vi "cluster_append.vi"(0 "magnitude value":dbl, 1 "phase value":dbl, 2 "Tx FFT mag":dbl, 3 "Tx FFT phase":dbl, 4 "shift value":dbl, 5 "Input Cluster":T1={"Magnitude meas."=[], "Phase meas."=[], "Shift meas."=[], "cw"=TRUE, "projections per image"=0, "ramp-up readouts"=0, "current sense type"="", "Number of pulses per image"=0, "Rotation enabled"=TRUE, "Rotary position"=[], "Baseline magnitude"=0.0, "Baseline phase"=0.0, "Wait readouts"=0, "Shift waveform type"="", "Shift enabled"=TRUE, "Time domain data"=[], "Motor pulse duration"=0.0, "Shift Amp pk"=0.0, "Shift DC offset"=0.0, "Notes"="", "Reconstructed image"=bytes[0], "Rotary encoder type"="", "Image start"=timestamp(0 s since 1904-01-01), "Image stop"=timestamp(0 s since 1904-01-01), "readouts per projection"=0, "Recon enabled"=FALSE, "Bidirectional shift"=FALSE, "Imager mode"="", "Shift delay"=0.0, "Shift frequency"=0.0, "Image time (calc)"=0.0, "Initial encoder position"=0.0, "Recon data"=[], "Trigger line values"=[], "Bed position"=0.0, "Sample image"=bytes[0], "Patch amplitude"=0.0, "Patch frequency"=0.0, "Patch phase"=0.0, "proj mag f2-f9"=[], "proj phase f2-f9"=[], "Tx waveform"=[], "Tx FFT mag"=[], "Tx FFT phase"=[], "Temps"=[]}, 7 "Rotary encoder":dbl, 9 "temps":dbl[](array[numeric]), 11 "Trigger line":i32, 14 "mag f2-f9":dbl[](array[numeric]), 15 "phase f2-f9":dbl[](array[numeric])) -> (19 "Output Cluster":T1={"Magnitude meas."=[], "Phase meas."=[], "Shift meas."=[], "cw"=TRUE, "projections per image"=0, "ramp-up readouts"=0, "current sense type"="", "Number of pulses per image"=0, "Rotation enabled"=TRUE, "Rotary position"=[], "Baseline magnitude"=0.0, "Baseline phase"=0.0, "Wait readouts"=0, "Shift waveform type"="", "Shift enabled"=TRUE, "Time domain data"=[], "Motor pulse duration"=0.0, "Shift Amp pk"=0.0, "Shift DC offset"=0.0, "Notes"="", "Reconstructed image"=bytes[0], "Rotary encoder type"="", "Image start"=timestamp(0 s since 1904-01-01), "Image stop"=timestamp(0 s since 1904-01-01), "readouts per projection"=0, "Recon enabled"=FALSE, "Bidirectional shift"=FALSE, "Imager mode"="", "Shift delay"=0.0, "Shift frequency"=0.0, "Image time (calc)"=0.0, "Initial encoder position"=0.0, "Recon data"=[], "Trigger line values"=[], "Bed position"=0.0, "Sample image"=bytes[0], "Patch amplitude"=0.0, "Patch frequency"=0.0, "Patch phase"=0.0, "proj mag f2-f9"=[], "proj phase f2-f9"=[], "Tx waveform"=[], "Tx FFT mag"=[], "Tx FFT phase"=[], "Temps"=[]})   [LabVIEW 2021]
panel:
  # "Append Values to Cluster arrays"
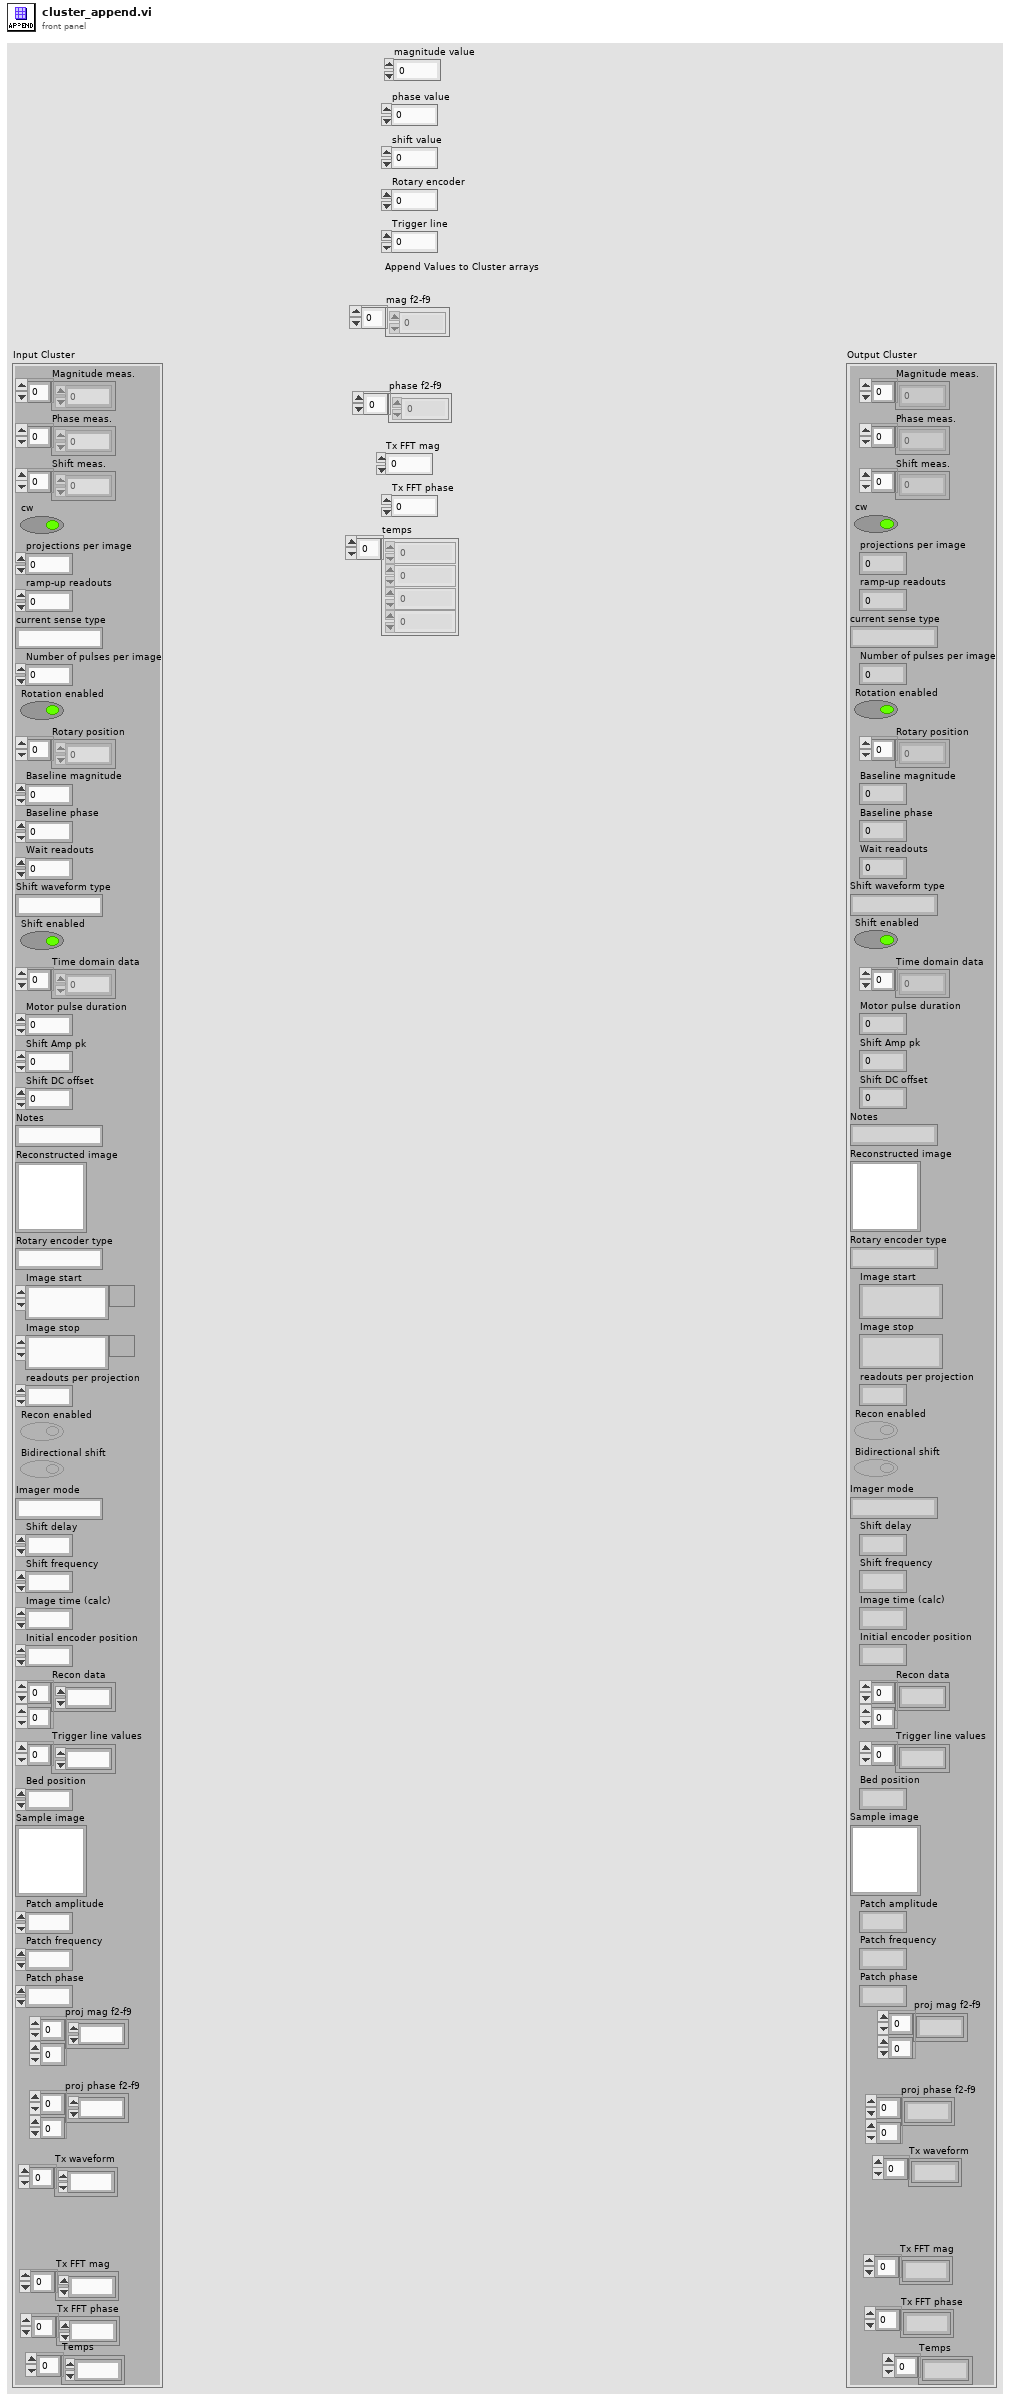
[diagram p1: front panel]
types:
  T1 = cluster{"Magnitude meas.":dbl[], "Phase meas.":dbl[], "Shift meas.":dbl[], "cw":bool, "projections per image":i32, "ramp-up readouts":i32, "current sense type":string, "Number of pulses per image":i32, "Rotation enabled":bool, "Rotary position":dbl[], "Baseline magnitude":dbl, "Baseline phase":dbl, "Wait readouts":i32, "Shift waveform type":string, "Shift enabled":bool, "Time domain data":dbl[], "Motor pulse duration":dbl, "Shift Amp pk":dbl, "Shift DC offset":dbl, "Notes":string, "Reconstructed image":picture, "Rotary encoder type":string, "Image start":timestamp, "Image stop":timestamp, "readouts per projection":i32, "Recon enabled":bool, "Bidirectional shift":bool, "Imager mode":string, "Shift delay":dbl, "Shift frequency":dbl, "Image time (calc)":dbl, "Initial encoder position":dbl, "Recon data":dbl[][], "Trigger line values":i32[], "Bed position":dbl, "Sample image":picture, "Patch amplitude":dbl, "Patch frequency":dbl, "Patch phase":dbl, "proj mag f2-f9":dbl[][], "proj phase f2-f9":dbl[][], "Tx waveform":dbl[], "Tx FFT mag":dbl[], "Tx FFT phase":dbl[], "Temps":dbl[]}
  T2 = cluster{"Magnitude meas.":dbl[], "Phase meas.":dbl[], "Shift meas.":dbl[], "cw":bool, "projections per image":i32, "ramp-up readouts":i32, "current sense type":string, "Number of pulses per image":i32, "Rotation enabled":bool, "Rotary position":dbl[], "Baseline magnitude":dbl, "Baseline phase":dbl, "Wait readouts":i32, "Shift waveform type":string, "Shift enabled":bool, "Time domain data":dbl[], "Motor pulse duration":dbl, "Shift start":dbl, "Shift stop":dbl, "Notes":string, "Reconstructed image":picture, "Rotary encoder type":string, "Image start":timestamp, "Image stop":timestamp, "readouts per projection":i32, "Recon enabled":bool, "Bidirectional shift":bool, "Imager mode":string, "Shift delay":dbl, "Shift frequency":dbl, "Image time (calc)":dbl, "Initial encoder position":dbl, "Recon data":dbl[][], "Trigger line values":i32[], "Bed position":dbl, "Sample image":picture, "Patch amplitude":dbl, "Patch frequency":dbl, "Patch phase":dbl, "proj mag f2-f9":dbl[][], "proj phase f2-f9":dbl[][], "Tx waveform":dbl[], "Tx FFT mag":dbl[], "Tx FFT phase":dbl[], "Temps":dbl[][]}
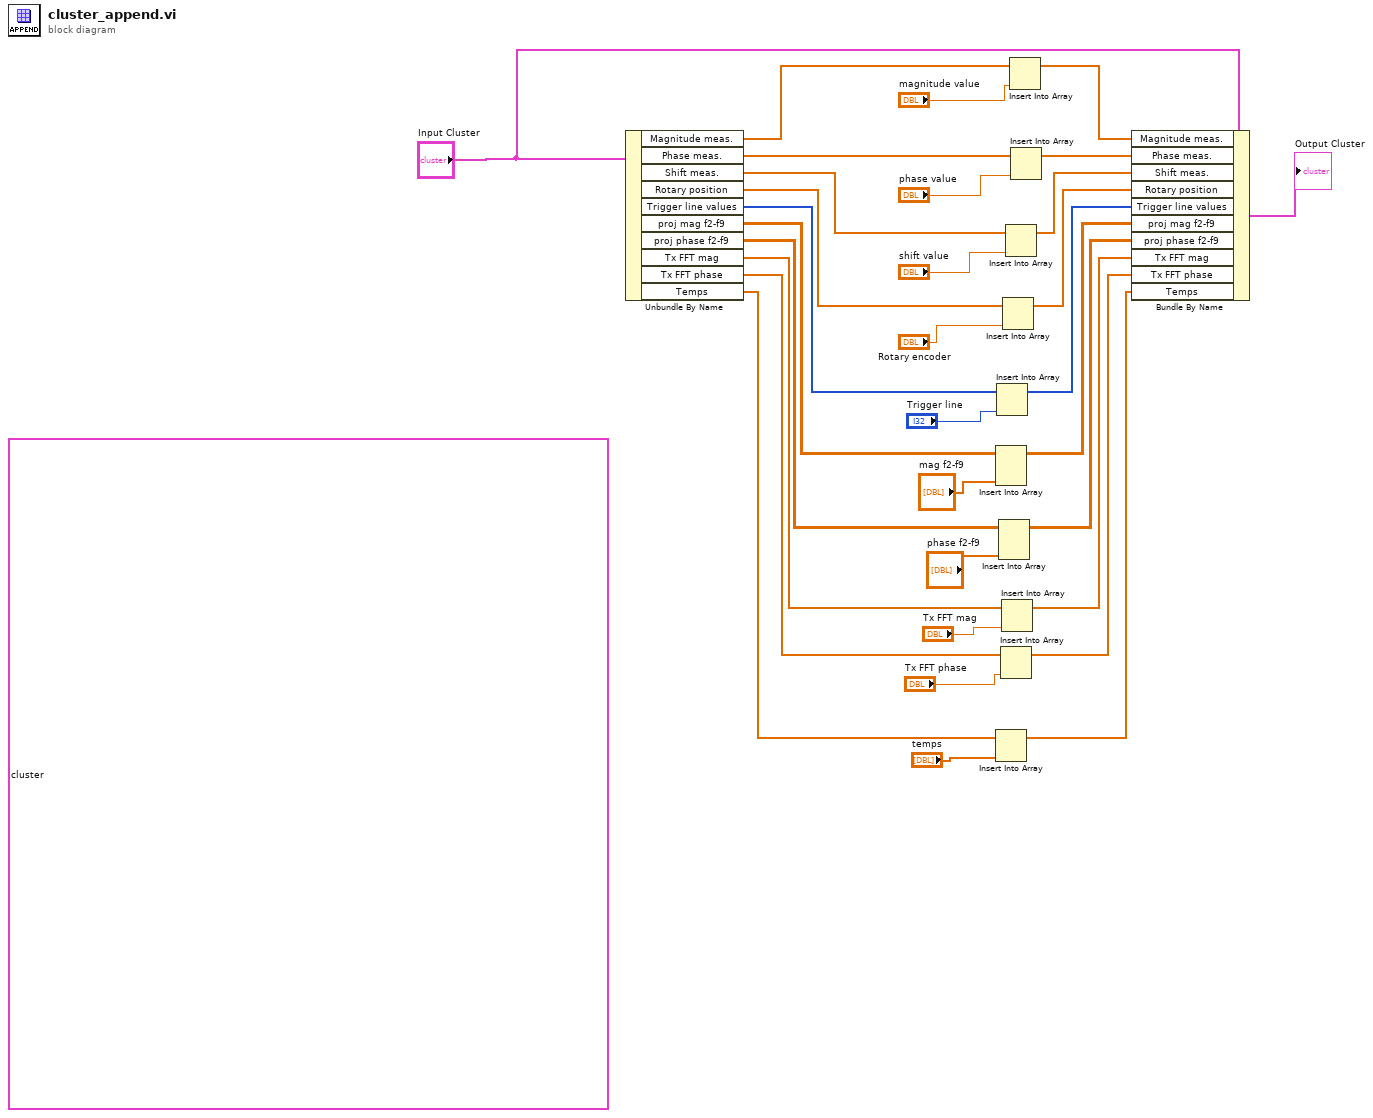
[diagram p0: block diagram]
diagram:
  (unwired) T2 {"Magnitude meas."=[], "Phase meas."=[], "Shift meas."=[], "cw"=TRUE, "projections per image"=0, "ramp-up readouts"=0, "current sense type"="", "Number of pulses per image"=0, "Rotation enabled"=TRUE, "Rotary position"=[], "Baseline magnitude"=0.0, "Baseline phase"=0.0, "Wait readouts"=0, "Shift waveform type"="", "Shift enabled"=TRUE, "Time domain data"=[], "Motor pulse duration"=0.0, "Shift start"=0.0, "Shift stop"=0.0, "Notes"="", "Reconstructed image"=bytes[0], "Rotary encoder type"="", "Image start"=timestamp(0 s since 1904-01-01), "Image stop"=timestamp(0 s since 1904-01-01), "readouts per projection"=0, "Recon enabled"=FALSE, "Bidirectional shift"=FALSE, "Imager mode"="", "Shift delay"=0.0, "Shift frequency"=0.0, "Image time (calc)"=0.0, "Initial encoder position"=0.0, "Recon data"=[], "Trigger line values"=[], "Bed position"=0.0, "Sample image"=bytes[0], "Patch amplitude"=0.0, "Patch frequency"=0.0, "Patch phase"=0.0, "proj mag f2-f9"=[], "proj phase f2-f9"=[], "Tx waveform"=[], "Tx FFT mag"=[], "Tx FFT phase"=[], "Temps"=[]}
  n1 = Unbundle By Name("Input Cluster") -> ("Magnitude meas."=w27:dbl[], "Phase meas."=w30:dbl[], "Shift meas."=w28:dbl[], "Rotary position"=w22:dbl[], "Trigger line values"=w20:i32[], "proj mag f2-f9"=w14:dbl[][], "proj phase f2-f9"=w11:dbl[][], "Tx FFT mag"=w9:dbl[], "Tx FFT phase"=w7:dbl[], "Temps"=w2:dbl[])
  n2 = Insert Into Array(array=w14, new element="mag f2-f9") -> (w13:dbl[][])  [unwired: 2 in]
  n3 = Insert Into Array(array=w2, new element="temps") -> (w1:dbl[])  [unwired: 1 in]
  n4 = Insert Into Array(array=w20, new element="Trigger line") -> (w18:i32[])  [unwired: 1 in]
  n5 = Insert Into Array(array=w11, new element="phase f2-f9") -> (w10:dbl[][])  [unwired: 2 in]
  n6 = Insert Into Array(array=w7, new element="Tx FFT phase") -> (w6:dbl[])  [unwired: 1 in]
  n7 = Insert Into Array(array=w9, new element="Tx FFT mag") -> (w8:dbl[])  [unwired: 1 in]
  n8 = Insert Into Array(array=w22, new element="Rotary encoder") -> (w23:dbl[])  [unwired: 1 in]
  n9 = Insert Into Array(array=w28, new element="shift value") -> (w24:dbl[])  [unwired: 1 in]
  n10 = Insert Into Array(array=w27, new element="magnitude value") -> (w26:dbl[])  [unwired: 1 in]
  n11 = Insert Into Array(array=w30, new element="phase value") -> (w25:dbl[])  [unwired: 1 in]
  n12 = Bundle By Name(cluster="Input Cluster", "Magnitude meas."=w26, "Phase meas."=w25, "Shift meas."=w24, "Rotary position"=w23, "Trigger line values"=w18, "proj mag f2-f9"=w13, "proj phase f2-f9"=w10, "Tx FFT mag"=w8, "Tx FFT phase"=w6, "Temps"=w1) -> (→"Output Cluster":T1)
